vi "Write Data.vi"(6 "chip select  (1st chip)":enum16{"1st chip", "2nd chip"}(ring), 8 "error in (no error)":errorcluster, 10 "character code":u8=97 format="%.0x", 11 "HD44780 in":refnum<class "HD44780.lvclass">) -> (0 "error out":errorcluster, 3 "HD44780 out":refnum<class "HD44780.lvclass">)   [LabVIEW 2017, in "HD44780.lvclass"]
uses:
  HD44780.lvclass
  HD44780.lvclass/HD44780.ctl
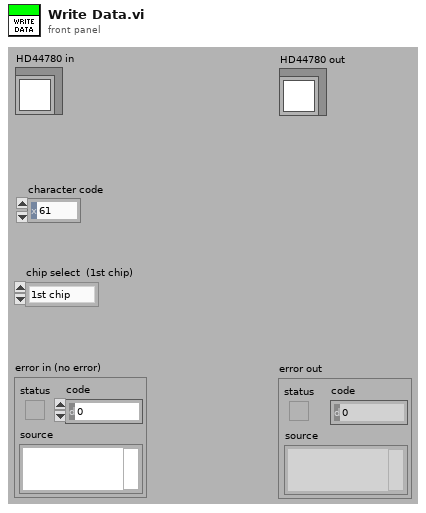
[diagram p1: front panel]
types:
  T1 = typedef "HD44780 Common.lvlib/cluster of class private data.ctl" = cluster{"FPGA VI Reference":refnum<k20>, "device index":i8, "screen size":T2, "font size":T3, "auto wrap":bool, "alignment":T4, "number of line":T5, "shift 0":i8, "entry mode 0":T6, "shift 1":i8, "entry mode 1":T6}
  T2 = typedef "HD44780 Common.lvlib/screen size.ctl" = enum8{"8x1", "8x2", "12x4", "16x1", "16x2", "16x4", "20x1", "20x2", "20x4", "24x1", "24x2", "40x2", "40x4"}
  T3 = typedef "HD44780 Common.lvlib/font size.ctl" = enum8{"5x8", "5x10"}
  T4 = typedef "HD44780 Common.lvlib/alignment.ctl" = enum16{"None", "Left", "Center", "Right"}
  T5 = typedef "HD44780 Common.lvlib/line number.ctl" = enum8{"1 line", "2 lines"}
  T6 = typedef "HD44780 Common.lvlib/entry mode.ctl" = enum8{"increment & no shift", "increment & shift", "decrement & no shift", "decrement & shift"}
  T7 = cluster{"FPGA VI Reference":refnum<k20>, "device index":i8, "screen size":enum8{"8x1", "8x2", "12x4", "16x1", "16x2", "16x4", "20x1", "20x2", "20x4", "24x1", "24x2", "40x2", "40x4"}, "font size":enum8{"5x8", "5x10"}, "auto wrap":bool, "alignment":enum16{"None", "Left", "Center", "Right"}, "number of line":enum8{"1 line", "2 lines"}, "shift 0":i8, "entry mode 0":enum8{"increment & no shift", "increment & shift", "decrement & no shift", "decrement & shift"}, "shift 1":i8, "entry mode 1":enum8{"increment & no shift", "increment & shift", "decrement & no shift", "decrement & shift"}}
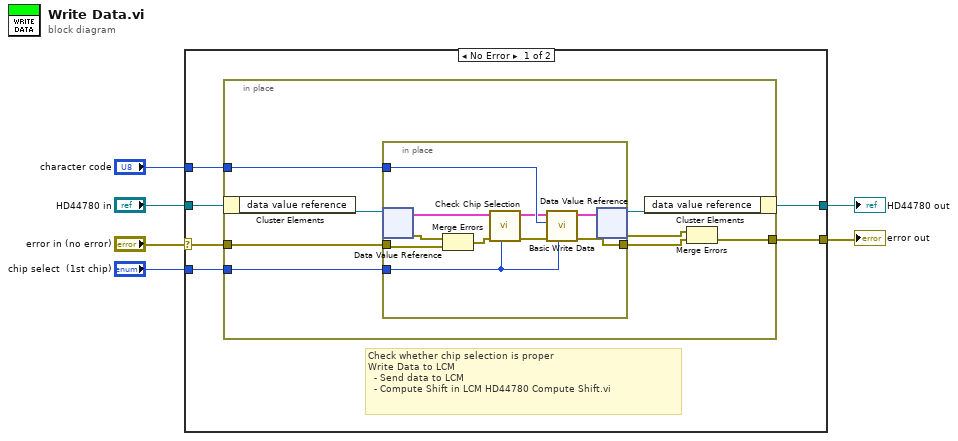
[diagram p0: block diagram]
diagram:
  n1 = case shown="No Error" "error in (no error)" {
    selector: "error in (no error)" -> [w8 w31]
    tunnel: "character code" -> [w12 _]
    tunnel: "chip select  (1st chip)" -> [w11 _]
    tunnel: "HD44780 in" -> [w10 w32]
    tunnel: [w9 w32] -> w3
    tunnel: [w7 w31] -> w1
    frame No Error {
      # "Check whether chip selection is proper\nWrite Data to LCM\n  - Send data to LCM\n  - Compute Shift in LCM HD44780 Compute Shift.vi"
      n2 = in-place {
        in-place-border: w12 -> [w20]
        in-place-border: w11 -> [w19]
        in-place-border: w8 -> [w18]
        in-place-border: [w13] -> w7
        n3 = in-place-cluster #1(w10) -> ("data value reference"=w17:refnum<data-value>)
        n4 = in-place {
          in-place-border: w20 -> [w30]
          in-place-border: w19 -> [w21]
          in-place-border: w18 -> [w27]
          in-place-border: [w28] -> w15
          n5 = in-place-dvr #2(w17) -> (w25:T1, w26:errorcluster)
          n6 = Merge Errors(w26, w27) -> (w24:errorcluster)
          n7 = call "Check Chip Selection.vi"("chip select"=w21, "error in (no error)"=w24, "cluster of private data in"=w25) -> ("error out"=w23:errorcluster, "cluster of private data out"=w22:T7)  [unwired: 7 in]
          n8 = call "Basic Write Data.vi"("chip select  (1st chip)"=w21, "error in (no error)"=w23, "character code"=w30, "cluster of private data in"=w22) -> ("error out"=w28:errorcluster, "cluster of private data out"=w29:T7)  [unwired: 6 in]
          n9 = in-place-dvr #2(w29) -> (w16:refnum<data-value>, w14:errorcluster)
        }
        n10 = in-place-cluster #1("data value reference"=w16) -> (w9:refnum<class "HD44780.lvclass">)
        n11 = Merge Errors(w14, w15) -> (w13:errorcluster)
      }
    }
    frame Error {
    }
  }
  "error out" <- w1
  "HD44780 out" <- w3
